vi "Load position from FEN.vi"(8 "error in (no error)":errorcluster, 11 "FEN string":string) -> (0 "error out":errorcluster, 2 "Move counter":u16, 3 "Position out":refnum<class "Position.lvclass">)   [LabVIEW 2015, in "Chesslib.lvlib" / "Position.lvclass"]
uses:
  Position.lvclass
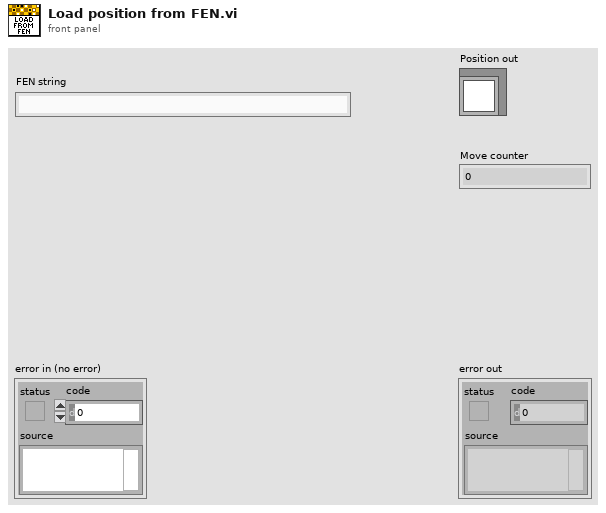
[diagram p1: front panel]
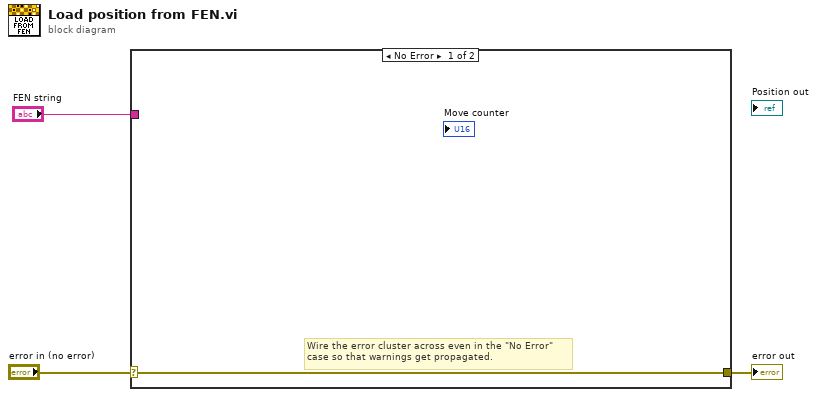
[diagram p0: block diagram]
diagram:
  n1 = case shown="No Error" "error in (no error)" {
    selector: "error in (no error)" -> [w4 w5]
    tunnel: [w4 w5] -> w2
    tunnel: "FEN string" -> [_ _]
    frame No Error {
      # "Wire the error cluster across even in the \"No Error\"\ncase so that warnings get propagated."
    }
    frame Error {
    }
  }
  "error out" <- w2
